vi "Update System Buttons.vi"(8 "System Button Refs":refnum<vi>[](array[refnum]), 9 "DAQ Rack Refs":refnum<vi>[](array[refnum]), 10 "System Index":i32, 11 "SubPanel in":refnum<vi>) -> ()   [LabVIEW 2019]
uses:
  Type Defs and Controls/System Button/System Button.xctl
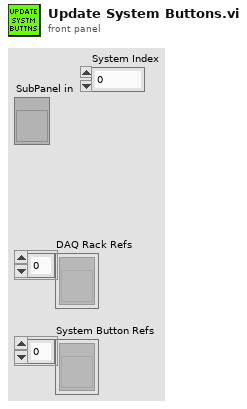
[diagram p1: front panel]
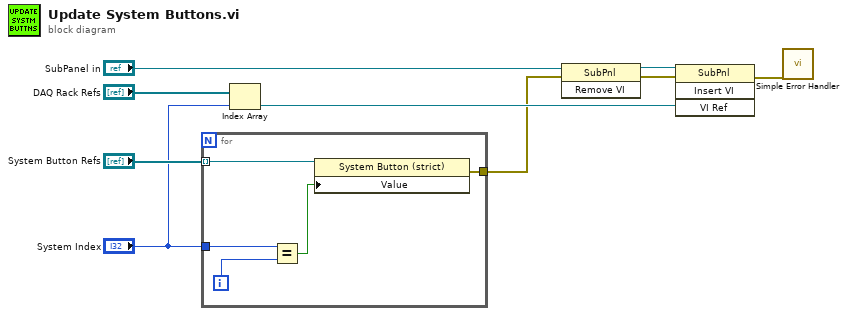
[diagram p0: block diagram]
diagram:
  n1 = for {
    tunnel: "System Button Refs" -> [w13] mode=indexing
    tunnel: "System Index" -> [w14]
    tunnel: [w11] -> w3
    i -> [w10]
    n2 = Equal?(x=w14, y=w10) -> (x = y?=w12:bool)
    n3 = property class="System Button (strict)"(reference=w13, "Value"=w12) -> (error out=w11:errorcluster)  [unwired: 1 in, 1 out]
  }
  n4 = Index Array(array="DAQ Rack Refs", index="System Index") -> (element=w8:refnum<vi>)
  n5 = invoke on="Invoke Node" class="SubPnl" method="Remove VI"(reference="SubPanel in", error in=w3) -> (reference out=w5:refnum<vi>, error out=w4:errorcluster)  [unwired: 1 in, 1 out]
  n6 = invoke on="Invoke Node" class="SubPnl" method="Insert VI"(reference=w5, error in=w4, "VI Ref"=w8) -> (error out=w2:errorcluster)  [unwired: 1 in, 3 out]
  n7 = call <vilib>:"Simple Error Handler.vi"("error in (no error)"=w2) -> ()  [unwired: 4 in, 5 out]
